vi "SECoP-TimeStamp.vi"() -> (3 "timestamp":dbl format="%#.3f")   [LabVIEW 2015, in "SECoP.lvlib"]
uses:
  SECoP.lvlib
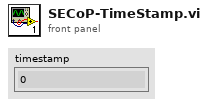
[diagram p1: front panel]
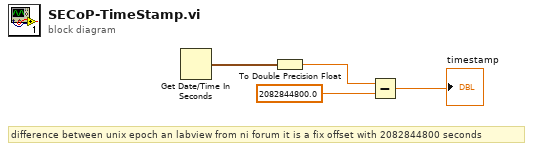
[diagram p0: block diagram]
diagram:
  # "difference between unix epoch an labview from ni forum it is a fix offset with 2082844800 seconds"
  n1 = Get Date/Time In Seconds() -> (seconds since 1Jan1904=w2:timestamp)
  n2 = To Double Precision Float(number=w2) -> (double precision float=w3:dbl)
  n3 = Subtract(x=w3, y=2082844800.0) -> (x-y=→"timestamp":dbl)
